vi "Create Data Store.vi"(8 "error in (no error)":errorcluster, 11 "Scan Driver.lvclass in":refnum<class "Scan Driver.lvclass">) -> (0 "error out":errorcluster, 3 "Scan Driver.lvclass out":refnum<class "Scan Driver.lvclass">)   [LabVIEW 2009, in "Scan Driver.lvclass"]
doc: "Initialize the internal Data Store. Call member Scanner instance to do the same."
uses:
  Scan Driver.lvclass
  Scan Driver.lvclass/Scan Driver.ctl
  Scanners/Scanner/Scanner.lvclass
  Readers/Reader/Reader.lvclass
  Data Processing/Aux Data Source/Aux Data Source.lvclass
  Instruments/Utility Classes/Readable/Data Point.ctl
  Instruments/Utility Classes/Readable/Readable.lvclass
  Instruments/Utility Classes/Readable/Data Channel.ctl
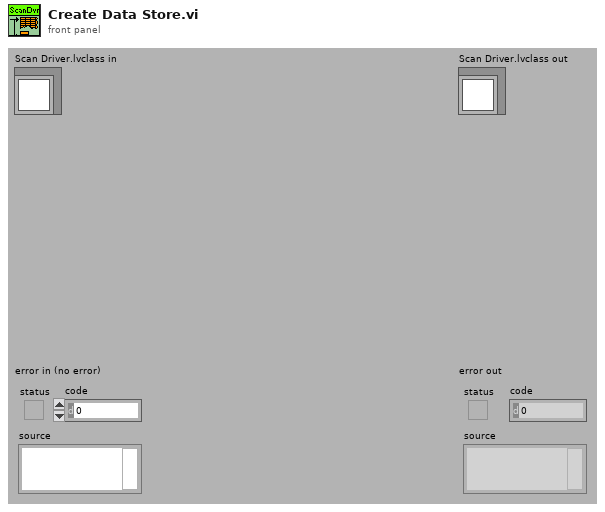
[diagram p1: front panel]
types:
  T1 = typedef "Readable.lvclass/Data Channel.ctl" = cluster{"Name":string, "Data Point":T2, "Unit":string}
  T2 = typedef "Readable.lvclass/Data Point.ctl" = dbl
  T3 = typedef "Readable.lvclass/Data Channels.ctl" = T1[]
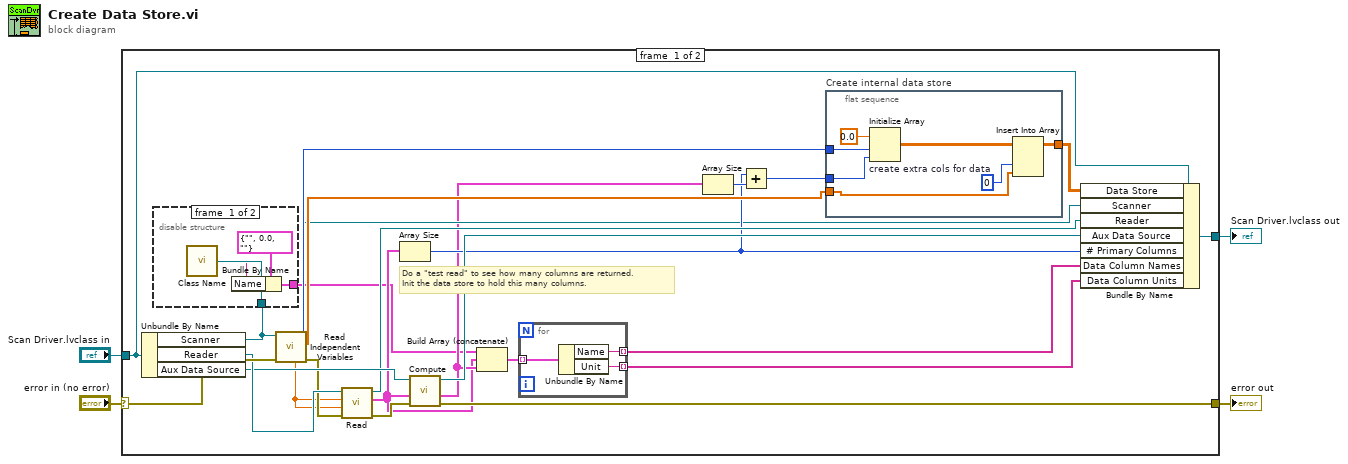
[diagram p0: block diagram]
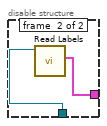
[diagram p2: hidden frame]
diagram:
  n1 = case shown="No Error" "error in (no error)" {
    selector: "error in (no error)" -> [w24 w46]
    tunnel: [w15 w46] -> w3
    tunnel: [w29 w47] -> w1
    tunnel: "Scan Driver.lvclass in" -> [w26 w47]
    frame #0 {
      # "Do a \"test read\" to see how many columns are returned.\nInit the data store to hold this many columns."
      n2 = Unbundle By Name(w26) -> ("Scanner"=w6:refnum<class "Scanner.lvclass">, "Reader"=w23:refnum<class "Reader.lvclass">, "Aux Data Source"=w22:refnum<class "Aux Data Source.lvclass">)
      n3 = disable-structure shown="Enabled" {
        disable-tunnel: [w32 w34] -> w7
        disable-tunnel: w6 -> [w31 w35]
        frame #0 {
          n4 = call "Class Name.vi"("LabVIEW Object"=w31) -> ("Classname"=w30:string)
          n5 = Bundle By Name(cluster=T1 {"Name"="", "Data Point"=0.0, "Unit"=""} ("Add'l Data Channels"), "Name"=w30) -> (w32:T1)
        }
        frame #1 {
          n6 = call-dynamic "Read Labels.vi"("Scanner in"=w35) -> ("Axis Label and Unit"=w34:T1)  [unwired: 8 in, 2 out]
        }
      }
      n7 = call-dynamic "Read Independent Variables.vi"("error in (no error)"=w24, "Scanner.lvclass in"=w6) -> ("error out"=w18:errorcluster, "size"=w25:i32, "Independent Variables"=w27:dbl[], "Scanner.lvclass out"=w13:refnum<class "Scanner.lvclass">, "min value"=w14:dbl)  [unwired: 5 out]
      n8 = call-dynamic "Read.vi"("error in (no error)"=w18, "Starting independent variable"=w14, "Current independent variable"=w14, "Reader in"=w23) -> ("error out"=w19:errorcluster, "Data Channels"=w11:T3, "Reader out"=w21:refnum<class "Reader.lvclass">)  [unwired: 5 in]
      n9 = Array Size(array=w11) -> (size(s)=w16:i32)
      n10 = call-dynamic "Compute.vi"("error in (no error)"=w19, "Data Channels"=w11, "Aux Data Source in"=w22) -> ("error out"=w15:errorcluster, "Add'l Data Channels"=w12:T3, "Aux Data Source out"=w20:refnum<class "Aux Data Source.lvclass">)  [unwired: 6 in]
      n11 = Build Array (concatenate)(w7, w11, w12) -> (w10:T3)
      n12 = for {
        tunnel: w10 -> [w38] mode=indexing
        tunnel: [w37] -> w9 mode=indexing
        tunnel: [w36] -> w8 mode=indexing
        n13 = Unbundle By Name(w38) -> ("Name"=w37:string, "Unit"=w36:string)
      }
      n14 = Array Size(array=w12) -> (size(s)=w17:i32)
      n15 = Add(x=w16, y=w17) -> (x+y=w5:i32)
      n16 = flat-sequence "Create internal data store" {
        tunnel: [w42] -> w28
        tunnel: w27 -> [w40]
        tunnel: w25 -> [w41]
        tunnel: w5 -> [w39]
        frame #0 {
          n17 = Initialize Array "create extra cols for data"(0.0, w41, w39) -> (w44:dbl[][])
          n18 = Insert Into Array(array=w44, index (col)=0 ("index (row)"), new element=w40) -> (w42:dbl[][])  [unwired: 1 in]
        }
      }
      n19 = Bundle By Name(cluster=w26, "Data Store"=w28, "Scanner"=w13, "Reader"=w21, "Aux Data Source"=w20, "# Primary Columns"=w16, "Data Column Names"=w9, "Data Column Units"=w8) -> (w29:refnum<class "Scan Driver.lvclass">)
    }
    frame #1 {
    }
  }
  "error out" <- w3
  "Scan Driver.lvclass out" <- w1
